vi "createCamera.vi"(8 "error in (no error)":errorcluster, 9 "machine name":string, 10 "Camera":string, 11 "NetworkWinX32 in":refnum<class "NetworkWinX32.lvclass">) -> (0 "error out":errorcluster, 3 "NetworkWinX32 out":refnum<class "NetworkWinX32.lvclass">)   [LabVIEW 2011, in "Hardware.lvlib" / "HWControllers.lvlib" / "NetworkWinX32.lvclass"]
uses:
  NetworkWinX32.lvclass
  Channels/Camera/WinX32_SA/WinX32Camera.lvclass
  Tools/Filing/FileSystem/FileSystem.lvclass
  NetworkWinX32.lvclass/NetworkWinX32.ctl
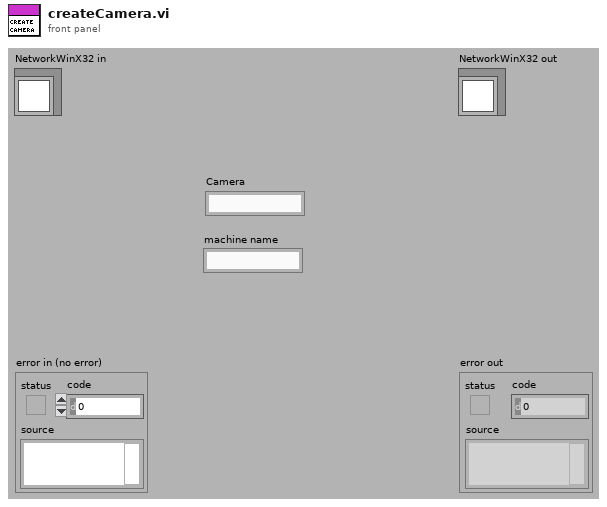
[diagram p1: front panel]
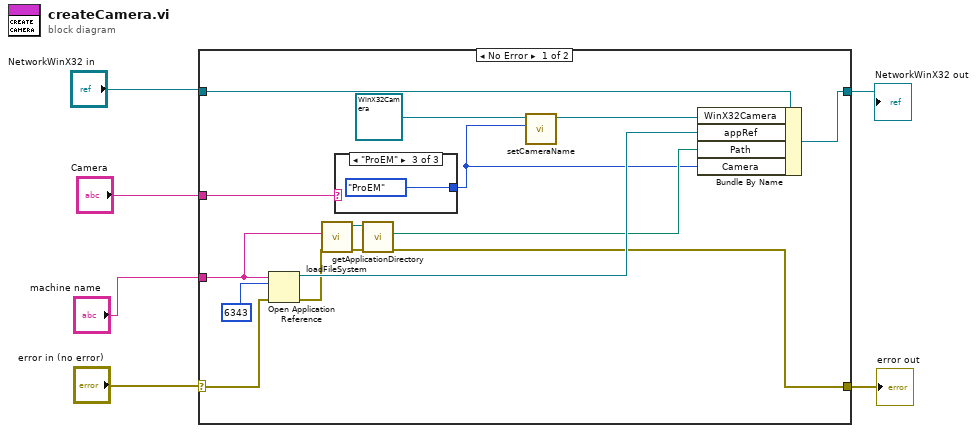
[diagram p0: block diagram]
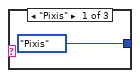
[diagram p2: hidden frame]
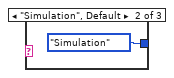
[diagram p3: hidden frame]
diagram:
  n1 = case shown="No Error" "error in (no error)" {
    selector: "error in (no error)" -> [w18 w25]
    tunnel: [w16 w26] -> w2
    tunnel: "NetworkWinX32 in" -> [w17 w26]
    tunnel: [w11 w25] -> w3
    tunnel: "machine name" -> [w19 _]
    tunnel: "Camera" -> [w10 _]
    frame No Error {
      n2 = Open Application Reference(8:w18, 10:6343, 11:w19) -> (0:w12:errorcluster, 3:w15:refnum<vi>)  [unwired: 1 in]
      n3 = call "loadFileSystem.vi"("error in (no error)"=w12, "computer name"=w19) -> ("error out"=w20:errorcluster, "FileSystem out"=w21:refnum<class "FileSystem.lvclass">)  [unwired: 8 in]
      n4 = case shown="\"ProEM\"" w10 {
        tunnel: [enum16{"Simulation", "Pixis", "ProEM"}."Pixis" ("Camera") enum16{"Simulation", "Pixis", "ProEM"}."Simulation" ("Camera") enum16{"Simulation", "Pixis", "ProEM"}."ProEM" ("Camera")] -> w7
        frame "Pixis" {
        }
        frame "Simulation", Default {
        }
        frame "ProEM" {
        }
      }
      n5 = call-dynamic "getApplicationDirectory.vi"("error in (no error)"=w20, "FileSystem.lvclass in"=w21) -> ("error out"=w11:errorcluster, "ApplicationDirectory"=w14:path)  [unwired: 7 in, 1 out]
      n6 = call "setCameraName.vi"("Camera"=w7, "WinX32Camera in"=refnum<class "WinX32Camera.lvclass"> refnum ("WinX32Camera.lvclass")) -> ("WinX32Camera out"=w9:refnum<class "WinX32Camera.lvclass">)  [unwired: 8 in, 1 out]
      n7 = Bundle By Name(cluster=w17, "WinX32Camera"=w9, "appRef"=w15, "Path"=w14, "Camera"=w7) -> (w16:refnum<class "NetworkWinX32.lvclass">)
    }
    frame Error {
    }
  }
  "error out" <- w3
  "NetworkWinX32 out" <- w2
